vi "Transition Measurements 1 chan.vi"(6 "percent level settings":T3={"method"=enum."auto select", "histogram size"=256, "histogram method"=enum."mode", "reserved"=1.0} {"reserved" format="%0.2f"}, 7 "edge number (1)":i32=1 min=1, 8 "error in (no error)":errorcluster, 9 "reference levels":T4={"high ref level"=90.0, "mid ref level"=50.0, "low ref level"=10.0, "ref units"=1} {"ref units" items=["absolute", "percent"]; "high ref level" format="%0.2f"; "low ref level" format="%0.2f"; "mid ref level" format="%0.2f"}, 10 "polarity (rising)":u16(ring)=1 items=["falling", "rising"], 11 "signal in":waveform(dbl)={"t0"=timestamp(0 s since 1904-01-01), "dt"=0.0, "Y"=[]}) -> (0 "error out":errorcluster, 1 "post-transition":T1, 2 "pre-transition":T1, 3 "transition duration":dbl, 4 "measurement info":T2 {"ref levels"."ref units" items=["absolute", "relative"]; "ref levels"."high ref level" format="%.2p"; "ref levels"."low ref level" format="%.2p"; "ref levels"."mid ref level" format="%.2p"; "end time" format="%.2p"; "start time" format="%.2p"}, 5 "slope":dbl)   [LabVIEW 2020, in "NI_MAPro.lvlib"]
doc: "Accepts an input signal of a single waveform or an array of waveforms and measures the transition duration (rise or fall time), slew rate, undershoot, and overshoot of a selected positive or negative transition in each waveform. Wire data to the <B>signal in</B> input to determine the polymorphic instance to use or manually select the instance."
uses:
  NI_MAPro.lvlib
  NI_MABase.lvlib
  <resource>/lvanlys.dll
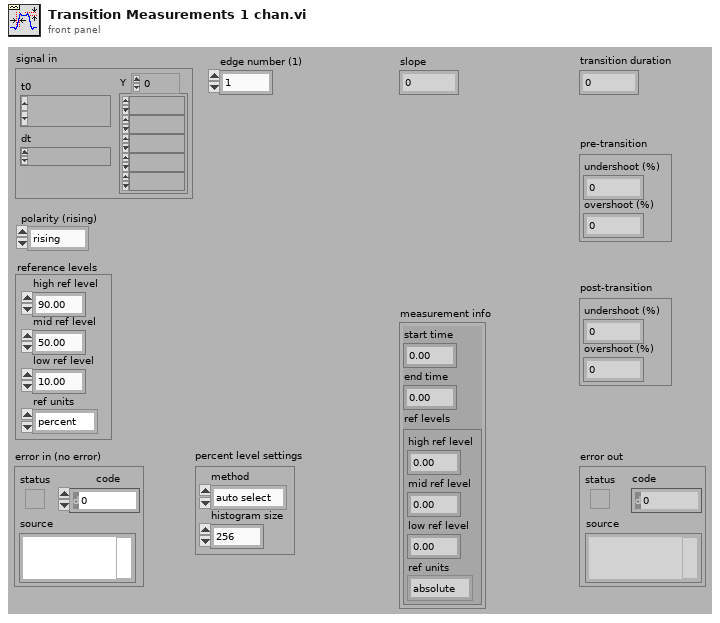
[diagram p1: front panel]
types:
  T1 = cluster{"undershoot (%)":dbl, "overshoot (%)":dbl}
  T2 = cluster{"start time":dbl, "end time":dbl, "ref levels":cluster{"high ref level":dbl, "mid ref level":dbl, "low ref level":dbl, "ref units":u16}}
  T3 = cluster{"method":enum32{"histogram", "peak", "auto select"}, "histogram size":i32, "histogram method":enum16{"mode"}, "reserved":dbl}
  T4 = cluster{"high ref level":dbl, "mid ref level":dbl, "low ref level":dbl, "ref units":u16}
  T5 = cluster{"PostUnderShoot":dbl, "PostOverShoot":dbl}
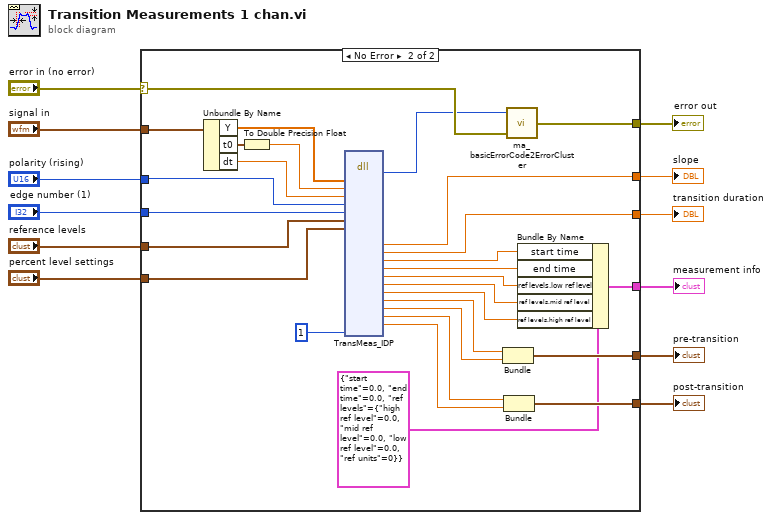
[diagram p0: block diagram]
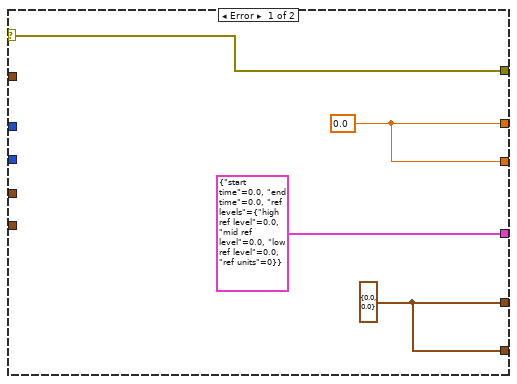
[diagram p2: hidden frame]
diagram:
  n1 = case shown="No Error" "error in (no error)" {
    selector: "error in (no error)" -> [w16 w43]
    tunnel: "polarity (rising)" -> [_ w38]
    tunnel: "reference levels" -> [_ w40]
    tunnel: "percent level settings" -> [_ w41]
    tunnel: "edge number (1)" -> [_ w39]
    tunnel: "signal in" -> [_ w44]
    tunnel: [T2 {"start time"=0.0, "end time"=0.0, "ref levels"={"high ref level"=0.0, "mid ref level"=0.0, "low ref level"=0.0, "ref units"=0}} ("measurement info") w35] -> w3
    tunnel: [w16 w42] -> w6
    tunnel: [w15 w36] -> w5
    tunnel: [w15 w37] -> w4
    tunnel: [w13 w34] -> w2
    tunnel: [w13 w33] -> w1
    frame Error {
      w13 = cluster{"PreUnderShoot":dbl, "PreOverShoot":dbl} {"PreUnderShoot"=0.0, "PreOverShoot"=0.0}
      w15 = 0.0 ("result")
    }
    frame No Error {
      n2 = Unbundle By Name(w44) -> ("Y"=w32:dbl[], "t0"=w31:timestamp, "dt"=w29:dbl)
      n3 = To Double Precision Float(number=w31) -> (double precision float=w30:dbl)
      n4 = dll-call lib="C:/Program Files (x86)/National Instruments/LabVIEW 2020/resource/lvanlys.*" fn="TransMeas_IDP"("xH"=w32, "Xo"=w30, "dx"=w29, "polarity"=w38, "edgeNum"=w39, "refLevel"=w40, "percentLevel"=w41, "newAlgorithm"=1) -> ("return type"=w17:i32, "slewRate"=w36:dbl, "transDuration"=w37:dbl, "startingTime"=w28:dbl, "endingTime"=w27:dbl, "lowRefLevel"=w26:dbl, "midRefLevel"=w25:dbl, "highRefLevel"=w24:dbl, "PreUnderShoot"=w22:dbl, "PreOverShoot"=w21:dbl, "PostUnderShoot"=w20:dbl, "PostOverShoot"=w19:dbl)  [unwired: 11 in, 15 out]
      n5 = Bundle("PreUnderShoot"=w22, "PreOverShoot"=w21) -> (w34:cluster{"PreUnderShoot":dbl, "PreOverShoot":dbl})  [unwired: 1 out]
      n6 = Bundle("PostUnderShoot"=w20, "PostOverShoot"=w19) -> (w33:T5)  [unwired: 1 out]
      n7 = call "ma_basicErrorCode2ErrorCluster.vi"("error in (no error)"=w43, "Error Code"=w17) -> ("error out"=w42:errorcluster)  [unwired: 1 in]
      n8 = Bundle By Name(cluster=T2 {"start time"=0.0, "end time"=0.0, "ref levels"={"high ref level"=0.0, "mid ref level"=0.0, "low ref level"=0.0, "ref units"=0}} ("measurement info"), "start time"=w28, "end time"=w27, "ref levels.low ref level"=w26, "ref levels.mid ref level"=w25, "ref levels.high ref level"=w24) -> (w35:T2)
    }
  }
  "slope" <- w5
  "transition duration" <- w4
  "measurement info" <- w3
  "error out" <- w6
  "post-transition" <- w1
  "pre-transition" <- w2
